vi "Enqueue Local Message.vi"(8 "error in":errorcluster, 9 "Data":variant, 10 "Message":string, 11 "Msg queue in":refnum<queue>) -> (0 "error out":errorcluster, 3 "queue out":refnum<queue>)   [LabVIEW 2019, in "Architecture.lvlib"]
doc: "This VI queues a message to a local message queue. Used to enqueue states in a single module state machine."
uses:
  Architecture.lvlib
  Typedefs/Message.ctl
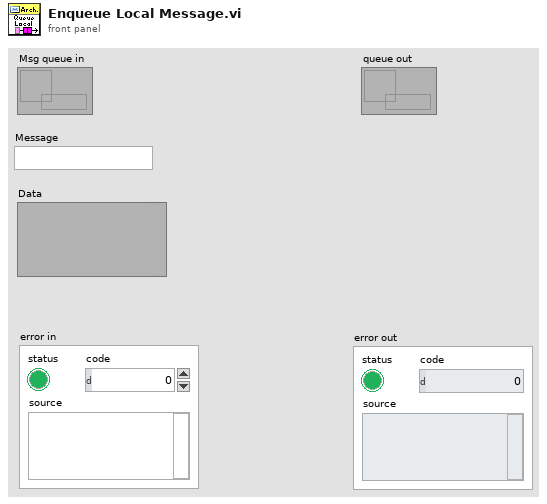
[diagram p1: front panel]
types:
  T1 = typedef "Architecture.lvlib/Message.ctl" = cluster{"Message":string, "Data":variant, "syn":bool}
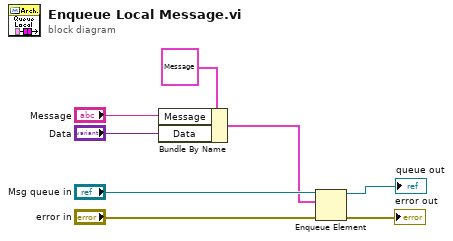
[diagram p0: block diagram]
diagram:
  n1 = Bundle By Name(cluster=T1 {"Message"="", "Data"=variant, "syn"=FALSE} ("element"), "Message"="Message", "Data"="Data") -> (w3:T1)
  n2 = Enqueue Element(queue="Msg queue in", element=w3, error in (no error)="error in") -> (queue out=→"queue out":refnum<queue>, error out=→"error out":errorcluster)  [unwired: 1 in, 1 out]
